vi "get_screenCenter.vi"(7 "use demo values?":bool, 8 "demo screen size":dbl[](array[numeric])=[640.0, 512.0], 11 "image":T1) -> (3 "screen center (px)":i32[](array[numeric]))   [LabVIEW 2015]
uses:
  <vilib>/vision/Image Controls.llb/IMAQ Image.ctl
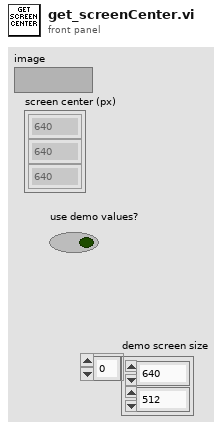
[diagram p1: front panel]
types:
  T1 = typedef "IMAQ Image.ctl" = refnum<image>
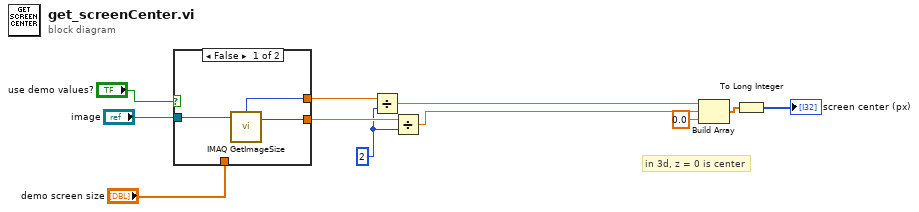
[diagram p0: block diagram]
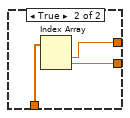
[diagram p2: hidden frame]
diagram:
  w5 = 2
  # "in 3d, z = 0 is center"
  n1 = case shown="False" "use demo values?" {
    tunnel: "image" -> [w14 _]
    tunnel: [w13 w16] -> w10
    tunnel: [w12 w15] -> w6
    tunnel: "demo screen size" -> [_ w17]
    frame False {
      n2 = call "IMAQ GetImageSize"("Image"=w14) -> ("Y Resolution"=w12:i32, "X Resolution"=w13:i32)  [unwired: 3 in, 1 out]
    }
    frame True {
      n3 = Index Array(array=w17) -> (element #1=w16:dbl, element #2=w15:dbl)  [unwired: 2 in]
    }
  }
  n4 = Divide(x=w10, y=w5) -> (x/y=w7:dbl)
  n5 = Divide(x=w6, y=w5) -> (x/y=w4:dbl)
  n6 = Build Array(w7, w4, 0.0 ("element")) -> (w9:dbl[])
  n7 = To Long Integer(number=w9) -> (32bit integer=→"screen center (px)":i32[])
